vi "CANOpen_Device Status .vi"(4 "Status NMT.Hardware Input.FIFO":refnum<k33>, 6 "Node IDs to Check":i16[](array[numeric]), 7 "interface object in":refnum<k20>, 8 "error in (no error)":errorcluster, 9 "Security Ref in":T10, 10 "Node States":u16[](array[numeric]), 11 "Nodes":T1[](array[typedef]) {"NMT"."Node init static SDO state" items=["start remote node"=1, "enter pre-operational"=128]; "NMT"."Node run state" items=["start remote node"=1, "stop remote node"=2, "enter pre-operational"=128, "reset node"=129, "reset communication"=130]; "Dynamic SDOs"."Sub-Index (0)" format="%.0x"; "Dynamic SDOs"."Object Index" format="%.0x"; "Dynamic SDOs"."Block Data" format="%.0x"; "RPDOs"."PDO Channel" items=["PDO 1", "PDO 2", "PDO 3", "PDO 4"]; "RPDOs"."Parameters"."Bit Offset" max=8 step=1; "RPDOs"."Parameters"."Byte Offset" max=8 step=1; "TPDOs"."PDO Channel" items=["PDO 1", "PDO 2", "PDO 3", "PDO 4"]; "TPDOs"."Parameters"."Bit Offset" max=8 step=1; "TPDOs"."Parameters"."Byte Offset" max=8 step=1; "SDOs"."Sub-Index (0)" format="%.0x"; "SDOs"."Object Index" format="%.0x"; "SDOs"."Block Data" format="%.0x"}) -> (0 "error out":errorcluster, 1 "Security Ref out":T10, 2 "Node States out":u16[](array[numeric]))   [LabVIEW 2021, in "CANOpen Addon Engine.lvlib"]
uses:
  CANOpen Addon Engine.lvlib
  Async VIs/CANOpen_Main/SubVIs/CANOpen_HB_NG_EM Refs.ctl
  CANOpen_Node Message Settings.ctl
  Shared/CANOpen_PDO Settings.ctl
  Shared/CANOpen_PDO Parameter Settings.ctl
  Shared/CANOpen_PDO Data Type.ctl
  System Explorer/SubVIs/CANopen Byte Order.ctl
  Shared/CANOpen_SDO Settings.ctl
  CANOpen_NMT Settings.ctl
  Async VIs/CANOpen_Main/SubVIs/CanOpen_NMT_Config.ctl
  Async VIs/CANOpen_Main/SubVIs/CanOpen_NMT_Static detect.ctl
  <vilib>/CANopenLib/CANOPEN.llb/CANopen Heartbeat State Read.vi
  <vilib>/CANopenLib/CANOPEN.llb/CANopen Node Guarding State Read.vi
  <vilib>/CANopenLib/CANOPEN.llb/CANopen Emergency Read.vi
  Shared/CANOpen Addon Shared.lvlib
  System Explorer/CANOpen Addon System Explorer.lvlib
panel:
  out "Time for read":u32
  # "LSB"
  # "MSB"
  # "LSB"
  # "MSB"
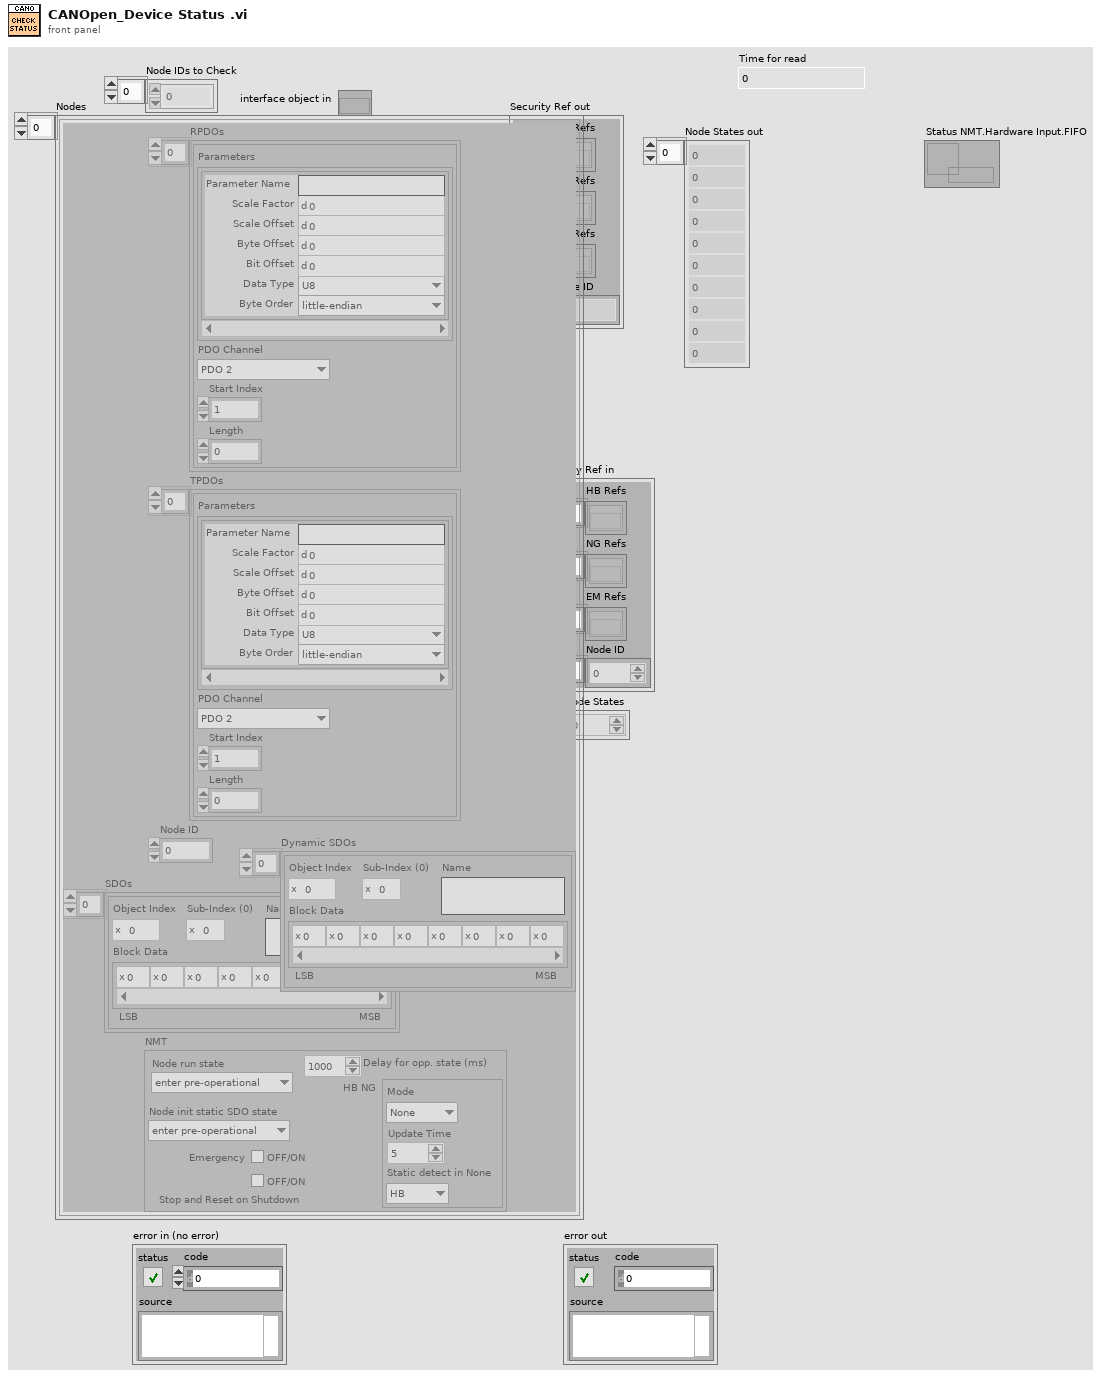
[diagram p1: front panel]
types:
  T1 = typedef "CANOpen Addon Engine.lvlib/CANOpen_Node Message Settings.ctl" = cluster{"RPDOs":T2[], "TPDOs":T2[], "Node ID":u8, "SDOs":T6[], "Dynamic SDOs":T6[], "NMT":T7}
  T2 = typedef "CANOpen Addon Shared.lvlib/CANOpen_PDO Settings.ctl" = cluster{"Parameters":T3[], "PDO Channel":u8, "Start Index":u32, "Length":u32}
  T3 = typedef "CANOpen Addon Shared.lvlib/CANOpen_PDO Parameter Settings.ctl" = cluster{"Parameter Name":string, "Scale Factor":dbl, "Scale Offset":dbl, "Byte Offset":u8, "Bit Offset":u8, "Data Type":T4, "Byte Order":T5}
  T4 = typedef "CANOpen Addon Shared.lvlib/CANOpen_PDO Data Type.ctl" = enum16{"U8", "U16", "U32", "I8", "I16", "I32", "Single", "Double", "Boolean"}
  T5 = typedef "CANOpen Addon System Explorer.lvlib/CANopen Byte Order.ctl" = enum16{"big-endian network order", "little-endian"}
  T6 = typedef "CANOpen Addon Shared.lvlib/CANOpen_SDO Settings.ctl" = cluster{"Object Index":u16, "Sub-Index (0)":u8, "Block Data":u8[], "Name":string}
  T7 = typedef "CANOpen Addon Engine.lvlib/CANOpen_NMT Settings.ctl" = cluster{"Node run state":u16, "Emergency":bool, "HB NG":T8, "Delay for opp. state (ms)":dbl, "Node init static SDO state":u16, "Stop and Reset on Shutdown":bool}
  T8 = typedef "CANOpen Addon Engine.lvlib/CanOpen_NMT_Config.ctl" = cluster{"Mode":T9, "Update Time":u16, "Static detect in None":T9}
  T9 = typedef "CANOpen Addon Engine.lvlib/CanOpen_NMT_Static detect.ctl" = enum16{"None", "HB", "NG"}
  T10 = typedef "CANOpen Addon Engine.lvlib/CANOpen_HB_NG_EM Refs.ctl" = cluster{"HB Refs":refnum<k20>[], "NG Refs":refnum<k20>[], "EM Refs":refnum<k20>[], "Node ID":u8[]}
  T11 = cluster{"error code":u16, "error register":u8, "manufacturer specific error field":u8[]}
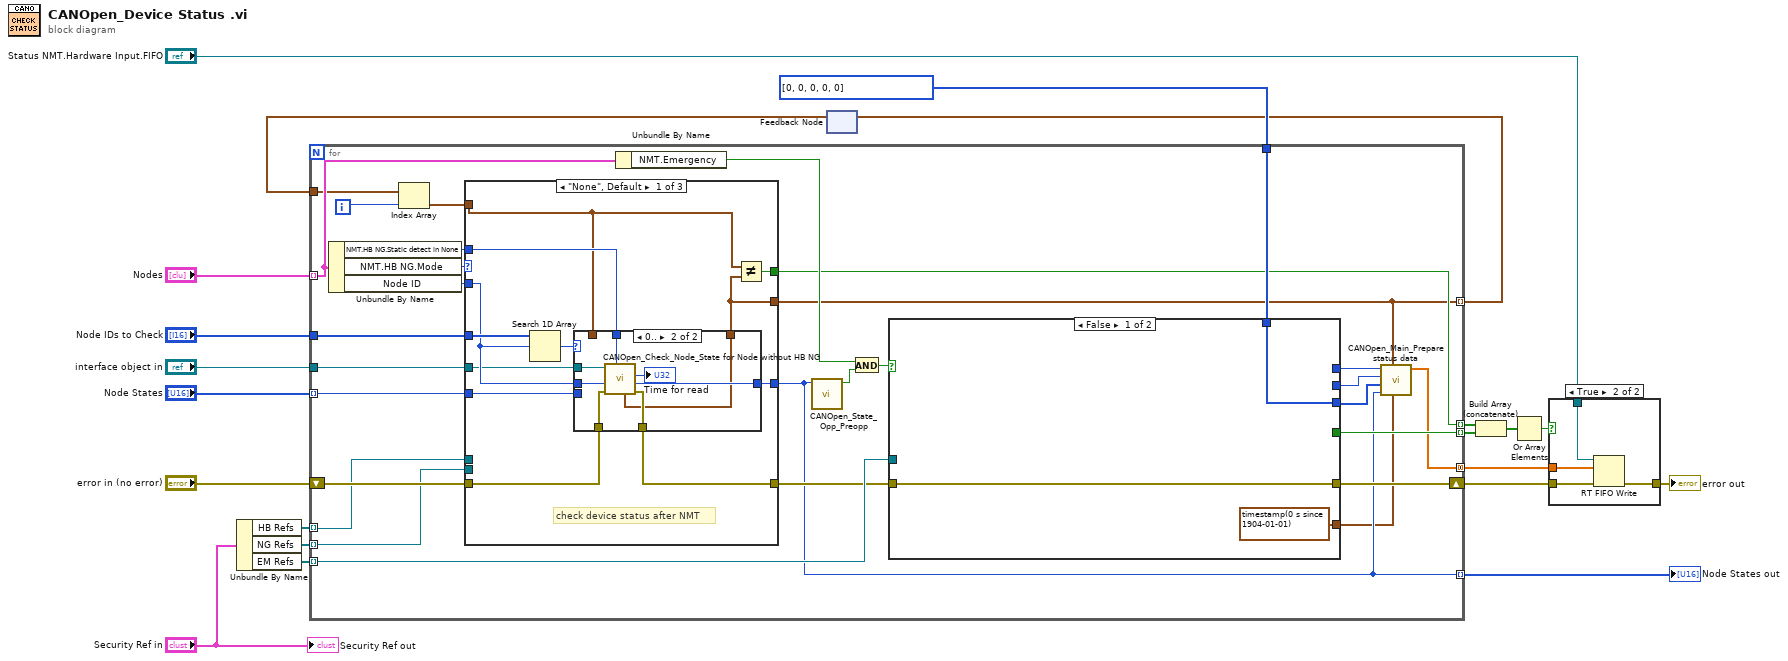
[diagram p0: block diagram]
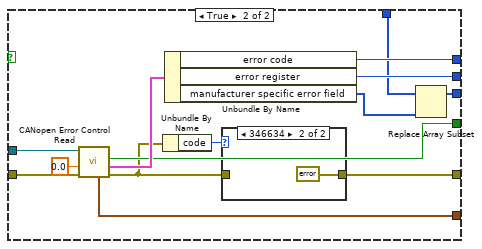
[diagram p3: hidden frame]
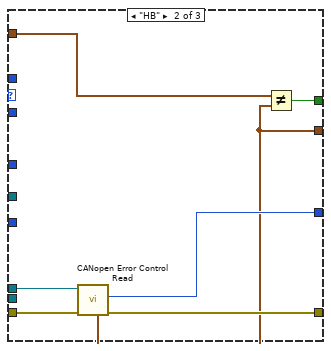
[diagram p6: hidden frame]
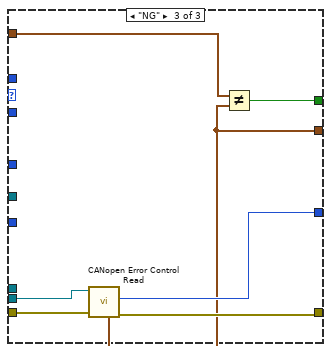
[diagram p7: hidden frame]
diagram:
  n1 = Unbundle By Name("Security Ref in") -> ("HB Refs"=w17:refnum<k20>[], "NG Refs"=w16:refnum<k20>[], "EM Refs"=w15:refnum<k20>[])
  n2 = feedback #1() -> (w1:timestamp[])  [unwired: 1 in]
  n3 = for {
    tunnel: "Nodes" -> [w49] mode=indexing
    tunnel: "Node States" -> [w42] mode=indexing
    shift-right: [w45] -> w9
    shift-left: "error in (no error)" -> [w46]
    tunnel: w17 -> [w44] mode=indexing
    tunnel: w16 -> [w43] mode=indexing
    tunnel: w15 -> [w48] mode=indexing
    tunnel: [w29] -> w7 mode=indexing
    tunnel: u8[] [0, 0, 0, 0, 0] ("manufacturer specific error field") -> [w41]
    tunnel: "Node IDs to Check" -> [w40]
    tunnel: "interface object in" -> [w38]
    tunnel: [w37] -> w5 mode=indexing
    tunnel: [w33] -> w6 mode=concatenating
    tunnel: [w27] -> w3 mode=indexing
    tunnel: [w25] -> w2 mode=indexing
    tunnel: w1 -> [w24]
    i -> [w23]
    n4 = Unbundle By Name(w49) -> ("NMT.HB NG.Static detect in None"=w28:T9, "NMT.HB NG.Mode"=w50:T9, "Node ID"=w39:u8)
    n5 = Index Array(array=w24, index=w23) -> (element=w22:timestamp)
    n6 = case shown="\"None\", Default" w50 {
      tunnel: w46 -> [w74 w99 w106]
      tunnel: [w73 w97 w104] -> w47
      tunnel: w44 -> [_ w98 _]
      tunnel: w43 -> [_ _ w105]
      tunnel: w42 -> [w76 _ _]
      tunnel: w40 -> [w81 _ _]
      tunnel: w39 -> [w79 _ _]
      tunnel: w38 -> [w78 _ _]
      tunnel: [w77 w95 w103] -> w29
      tunnel: w28 -> [w75 _ _]
      tunnel: [w72 w96 w102] -> w27
      tunnel: [w71 w93 w101] -> w25
      tunnel: w22 -> [w70 w94 w100]
      frame "None", Default {
        # "check device status after NMT"
        n7 = Search 1D Array(1D array=w81, element=w79) -> (index of element=w80:i32)  [unwired: 1 in]
        n8 = case shown="0.." w80 {
          tunnel: w79 -> [_ w92]
          tunnel: [w84 w91] -> w77
          tunnel: w74 -> [w83 w90]
          tunnel: w78 -> [_ w89]
          tunnel: w76 -> [w84 _]
          tunnel: w75 -> [_ w88]
          tunnel: [w83 w87] -> w73
          tunnel: [w82 w86] -> w71
          tunnel: w70 -> [w82 _]
          frame -1, Default {
          }
          frame 0.. {
            n9 = call "CANOpen_Check_Node_State for Node without HB NG.vi"("State detect in None"=w88, "error in"=w90, "Node ID"=w92, "interface object in"=w89) -> ("error out"=w87:errorcluster, "Last State"=w91:u16, "Time for read"=→"Time for read":u32, "timestamp"=w86:timestamp)  [unwired: 4 in]
          }
        }
        n10 = Not Equal?(x=w70, y=w71) -> (x != y?=w72:bool)
      }
      frame "HB" {
        n11 = call-poly <vilib>:"CANopen Error Control Read.vi"("error in (no error)"=w99, "heartbeat object in"=w98) -> ("error out"=w97:errorcluster, "state"=w95:u16, "timestamp"=w93:timestamp)  [unwired: 6 in, 1 out]
        n12 = Not Equal?(x=w94, y=w93) -> (x != y?=w96:bool)
      }
      frame "NG" {
        n13 = call-poly <vilib>:"CANopen Error Control Read.vi"("error in (no error)"=w106, "node guarding object in"=w105) -> ("error out"=w104:errorcluster, "state"=w103:u16, "timestamp"=w101:timestamp)  [unwired: 6 in, 1 out]
        n14 = Not Equal?(x=w100, y=w101) -> (x != y?=w102:bool)
      }
    }
    n15 = Unbundle By Name(w49) -> ("NMT.Emergency"=w36:bool)
    n16 = call "CANOpen_State_Opp_Preopp.vi"("state"=w29) -> ("Active"=w35:bool)  [unwired: 10 in]
    n17 = And(x=w36, y=w35) -> (x .and. y?=w34:bool)
    n18 = case shown="False" w34 {
      tunnel: w48 -> [_ w67]
      tunnel: w47 -> [w53 w66]
      tunnel: [w53 w55] -> w45
      tunnel: [timestamp(0 s since 1904-01-01) ("timestamp") w64] -> w26
      tunnel: [_ w62] -> w32
      tunnel: [_ w61] -> w31
      tunnel: [w52 w58] -> w30
      tunnel: w41 -> [w52 w60]
      tunnel: [_ w57] -> w37
      frame False {
      }
      frame True {
        n19 = call-poly <vilib>:"CANopen Error Control Read.vi"("error in (no error)"=w66, "timeout (0s)"=0.0, "emergency object in"=w67) -> ("error out"=w54:errorcluster, "emergency message"=w63:T11, "new message?"=w57:bool, "timestamp"=w64:timestamp)  [unwired: 4 in, 1 out]
        n20 = Unbundle By Name(w54) -> ("code"=w56:i32)
        n21 = Unbundle By Name(w63) -> ("error code"=w62:u16, "error register"=w61:u8, "manufacturer specific error field"=w59:u8[])
        n22 = case shown="346634" w56 {
          tunnel: [w68 errorcluster {"status"=FALSE, "code"=0, "source"=""} ("error out")] -> w55
          tunnel: w54 -> [w68 _]
          frame 0, Default {
          }
          frame 346634 {
          }
        }
        n23 = Replace Array Subset(array=w60, new element=w59) -> (w58:u8[])  [unwired: 1 in]
      }
    }
    n24 = call "CANOpen_Main_Prepare status data.vi"("EM timestamp"=w26, "timestamp"=w25, "state"=w29, "manufacturer specific error field"=w30, "EM Error Register"=w31, "EM Error Code"=w32) -> ("element"=w33:dbl[])  [unwired: 5 in]
  }
  "Node States out" <- w7
  n25 = feedback-in #1(w2) -> ()
  n26 = Build Array (concatenate)(w3, w5) -> (w4:bool[])
  n27 = Or Array Elements(Boolean array=w4) -> (logical OR=w8:bool)
  n28 = case shown="True" w8 {
    tunnel: "Status NMT.Hardware Input.FIFO" -> [_ w111]
    tunnel: [w107 w110] -> w10
    tunnel: w9 -> [w107 w109]
    tunnel: w6 -> [_ w108]
    frame False {
    }
    frame True {
      n29 = RT FIFO Write(0:w111, 1:w108, 3:w109) -> (11:w110:errorcluster)  [unwired: 2 in, 3 out]
    }
  }
  "error out" <- w10
  "Security Ref out" <- "Security Ref in"
